vi "CompileData.vi"(0 "refnum in":refnum<file>, 1 "Tank Pressure (Torr)":string, 3 "Middle":bool, 4 "Laser Power (W)":dbl, 5 "error in":errorcluster, 6 "Cryostat Temp (K)":dbl, 7 "Low Resistor":dbl, 8 "High Resistor":dbl, 9 "Ch. A (W)":string, 10 "Top":bool caption="Top Level", 11 "Bottom":bool, 12 "Cell Temp (K)":dbl, 13 "Ch. B (W)":string, 15 "Incident":dbl, 17 "Liquid Level":dbl, 18 "Detected":dbl) -> (14 "refnum out":refnum<file>, 19 "error out":errorcluster)   [LabVIEW 2018]
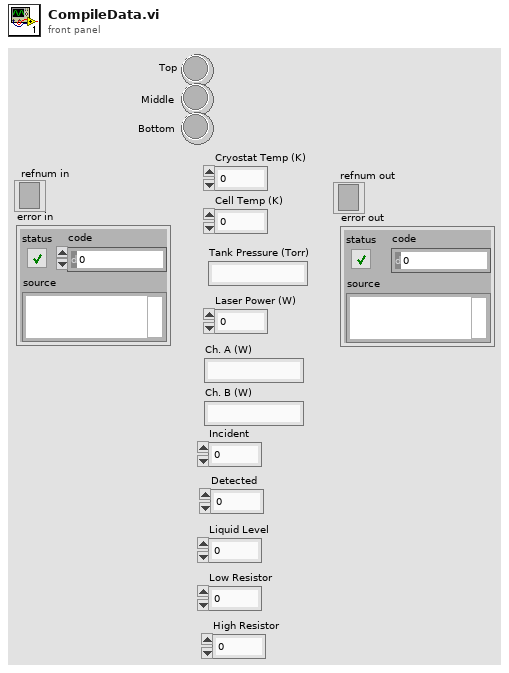
[diagram p1: front panel]
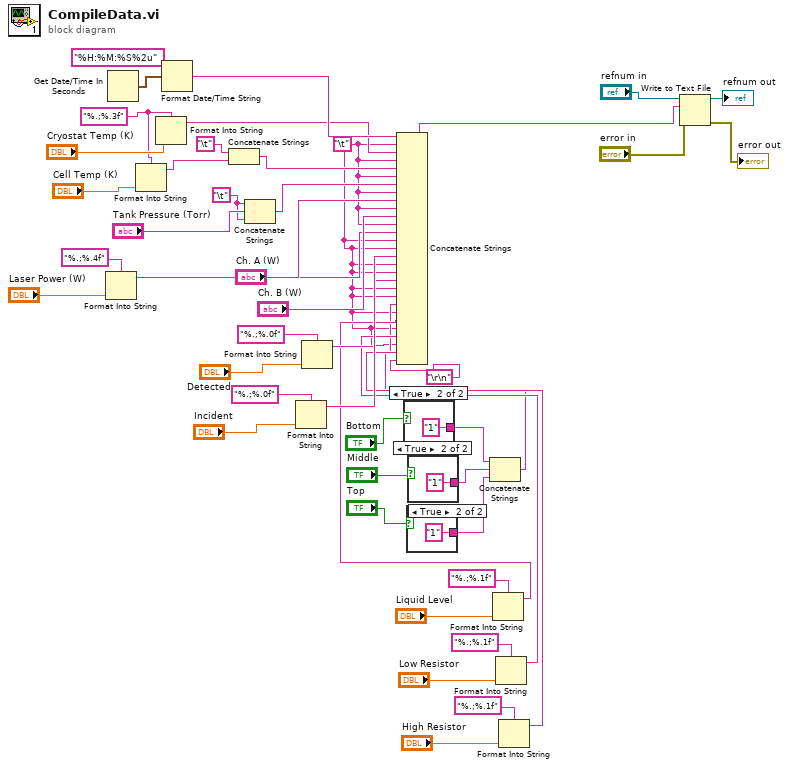
[diagram p0: block diagram]
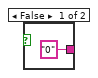
[diagram p2: hidden frame]
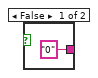
[diagram p3: hidden frame]
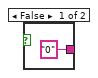
[diagram p4: hidden frame]
diagram:
  w29 = "\t"
  w1 = "\t"
  w26 = "%.;%.3f" ("format string")
  n1 = Format Into String(format string="%.;%.4f", "Laser Power (W)") -> (resulting string=w24:string)  [unwired: 2 in, 1 out]
  n2 = Get Date/Time In Seconds() -> (seconds since 1Jan1904=w46:timestamp)
  n3 = Format Into String(format string=w26, "Cell Temp (K)") -> (resulting string=w33:string)  [unwired: 2 in, 1 out]
  n4 = Format Into String(format string=w26, "Cryostat Temp (K)") -> (resulting string=w44:string)  [unwired: 2 in, 1 out]
  n5 = Format Date/Time String(time format string (%c)="%H:%M:%S%2u", seconds (now)=w46) -> (date/time string=w45:string)  [unwired: 1 in]
  n6 = Concatenate Strings("\t", w33) -> (w32:string)
  n7 = Concatenate Strings(w29, "Tank Pressure (Torr)", w29) -> (w30:string)
  n8 = Format Into String(format string="%.;%.0f", "Incident") -> (resulting string=w20:string)  [unwired: 2 in, 1 out]
  n9 = Format Into String(format string="%.;%.0f", "Detected") -> (resulting string=w19:string)  [unwired: 2 in, 1 out]
  n10 = case shown="True" "Bottom" {
    tunnel: ["0" ("string") "1" ("string")] -> w17
    frame False {
    }
    frame True {
    }
  }
  n11 = case shown="True" "Top" {
    tunnel: ["0" ("string") "1" ("string")] -> w13
    frame False {
    }
    frame True {
    }
  }
  n12 = case shown="True" "Middle" {
    tunnel: ["0" ("string") "1" ("string")] -> w14
    frame False {
    }
    frame True {
    }
  }
  n13 = Concatenate Strings(w17, w14, w13) -> (w2:string)
  n14 = Format Into String(format string="%.;%.1f", "Liquid Level") -> (resulting string=w3:string)  [unwired: 2 in, 1 out]
  n15 = Format Into String(format string="%.;%.1f", "Low Resistor") -> (resulting string=w4:string)  [unwired: 2 in, 1 out]
  n16 = Format Into String(format string="%.;%.1f", "High Resistor") -> (resulting string=w5:string)  [unwired: 2 in, 1 out]
  n17 = Concatenate Strings(w45, w1, w44, w1, w32, w1, w30, w1, "Ch. A (W)", w1, "Ch. B (W)", w1, w24, w1, w1, w20, w1, w1, w19, w1, w1, w2, w1, w3, w1, w4, w1, w5, "\r\n") -> (w43:string)
  n18 = Write to Text File(file (use dialog)="refnum in", text=w43, error in="error in") -> (refnum out=→"refnum out":refnum<file>, error out=→"error out":errorcluster)  [unwired: 1 in, 1 out]
